vi "GPOCT_Close.vi"(8 "error in (no error)":errorcluster, 11 "path in":path) -> (0 "error out":errorcluster)   [LabVIEW 2016]
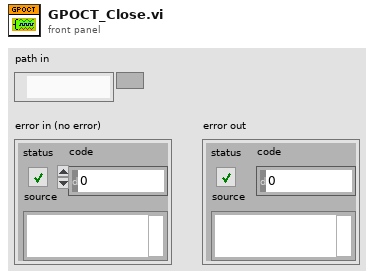
[diagram p1: front panel]
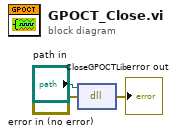
[diagram p0: block diagram]
diagram:
  n1 = dll-call lib="C:/Users/Mikael/Documents/Visual Studio 2015/Projects/GPOCT/x64/Release/GPOCT.dll" fn="CloseGPOCTLib"(path in="path in", error in="error in (no error)") -> (error out=→"error out":errorcluster)  [unwired: 2 in, 1 out]
